vi "发送.vi"() -> ()   [LabVIEW 2018]
panel:
  out "F-格式字符串":string
  out "长度 2":i32
  in  "客户端关闭":string="客户端VI关闭了连接。"
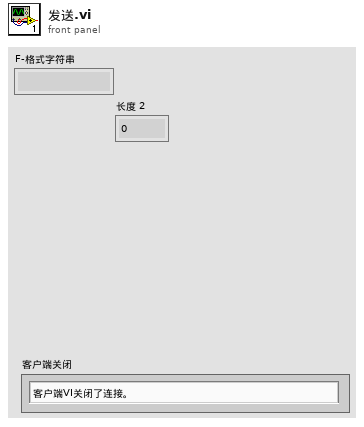
[diagram p1: front panel]
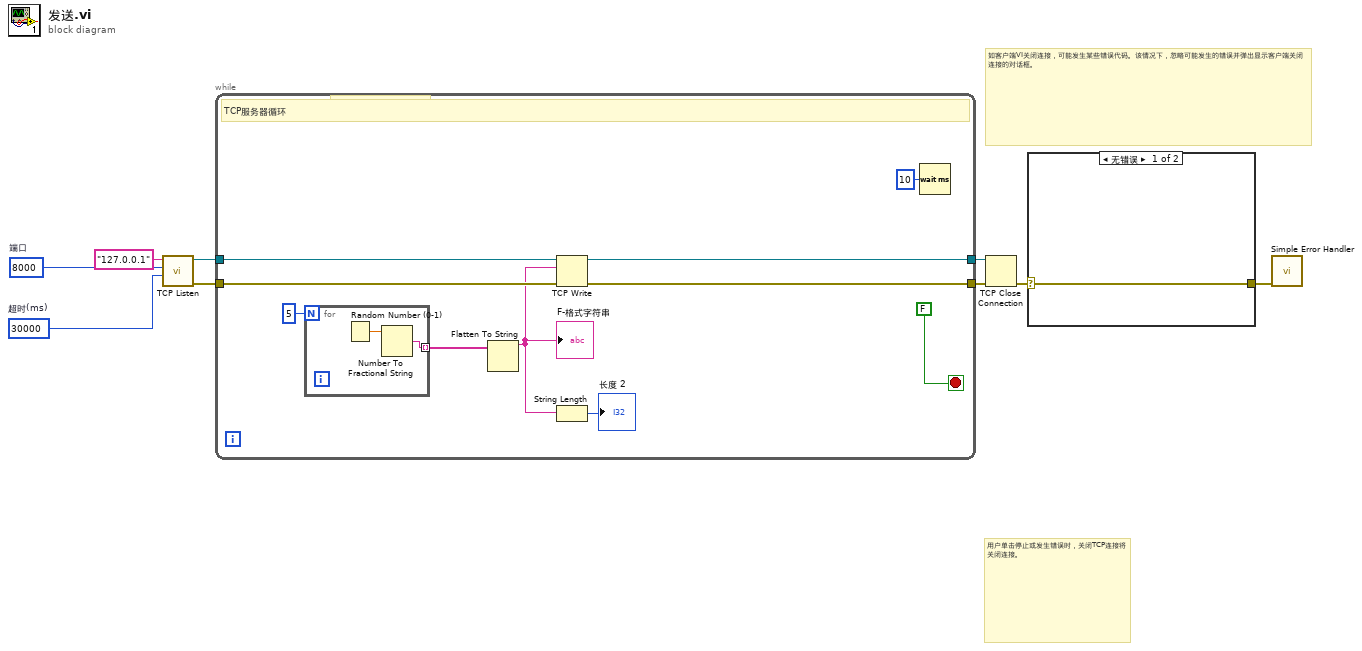
[diagram p0: block diagram]
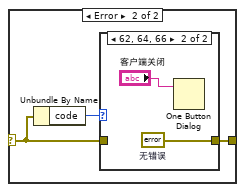
[diagram p2: hidden frame]
diagram:
  w4 = u16 8000  # 端口
  w5 = 30000  # 超时(ms)
  # "这个程序是服务端"
  # "用户单击停止或发生错误时，关闭TCP连接将关闭连接。"
  # "如客户端VI关闭连接，可能发生某些错误代码。该情况下，忽略可能发生的错误并弹出显示客户端关闭连接的对话框。"
  n1 = call <vilib>:"TCP Listen.vi"("timeout ms (wait forever: -1)"=w5, "port"=w4, "service name"="127.0.0.1") -> ("error out"=w6:errorcluster, "connection ID"=w7:refnum<k5>)  [unwired: 4 in, 3 out]
  n2 = while {
    tunnel: w7 -> [w18]
    tunnel: w6 -> [w17]
    tunnel: [w14] -> w3
    tunnel: [w15] -> w2
    stop <- FALSE stop-if-true
    # "TCP服务器循环"
    n3 = for {
      N: 5 -> [_]
      tunnel: [w20] -> w12 mode=indexing
      n4 = Random Number (0-1)() -> (number: 0 to 1=w21:dbl)
      n5 = Number To Fractional String(number=w21) -> (F-format string=w20:string)  [unwired: 3 in]
    }
    n6 = Flatten To String(anything=w12) -> (data string=w10:string)  [unwired: 3 in, 2 out]
    "F-格式字符串" <- w10
    n7 = TCP Write(connection ID=w18, data in=w10, error in (no error)=w17) -> (connection ID out=w14:refnum<k5>, error out=w15:errorcluster)  [unwired: 2 out]
    n8 = String Length(string=w10) -> (length=→"长度 2":i32)
    n9 = Wait (ms)(milliseconds to wait=u32 10) -> ()  [unwired: 1 out]
  }
  n10 = TCP Close Connection(connection ID=w3, error in (no error)=w2) -> (error out=w9:errorcluster)  [unwired: 2 out]
  n11 = case shown="无错误" w9 {
    selector: w9 -> [w22 w24]
    tunnel: [w22 w23] -> w8
    frame No Error {
    }
    frame Error {
      n12 = Unbundle By Name(w24) -> ("code"=w25:i32)
      n13 = case shown="62, 64, 66" w25 {
        tunnel: w24 -> [w26 _]
        tunnel: [w26 w28] -> w23
        frame Default {
        }
        frame 62, 64, 66 {
          w28 = errorcluster {"status"=FALSE, "code"=0, "source"=""}  # 无错误
          n14 = One Button Dialog(message="客户端关闭") -> ()  [unwired: 1 in, 1 out]
        }
      }
    }
  }
  n15 = call <vilib>:"Simple Error Handler.vi"("error in (no error)"=w8) -> ()  [unwired: 1 in, 8 out]
